vi "Setup NI cDAQ-9188.vi"(8 "error in":errorcluster, 9 "Samples per Channel":i32=100, 10 "Sample Rate":dbl=100000.0, 11 "Physical Channels":string) -> (0 "error out":errorcluster, 2 "Counter Task":refnum<k21>, 3 "AI Voltage Task":refnum<k21>)   [LabVIEW 2013, in "Breakdown Acoustics Controls.lvlib"]
uses:
  <vilib>/DAQmx/create/channels.llb/DAQmx Create Channel (AI-Voltage-Basic).vi
  <vilib>/DAQmx/configure/timing.llb/DAQmx Timing (Sample Clock).vi
  <vilib>/DAQmx/create/channels.llb/DAQmx Create Channel (CO-Pulse Generation-Frequency).vi
  <vilib>/DAQmx/configure/timing.llb/DAQmx Timing (Implicit).vi
  <vilib>/DAQmx/configure/trigger.llb/DAQmx Start Trigger (Digital Edge).vi
  Breakdown Acoustics Controls.lvlib
  <resource>/objmgr/daqmx.rc
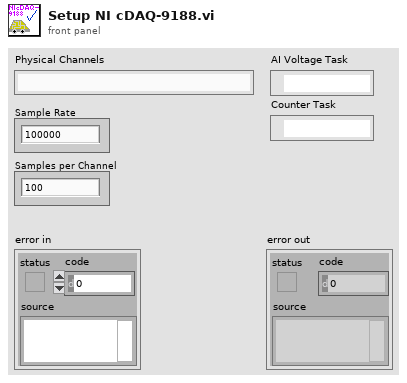
[diagram p1: front panel]
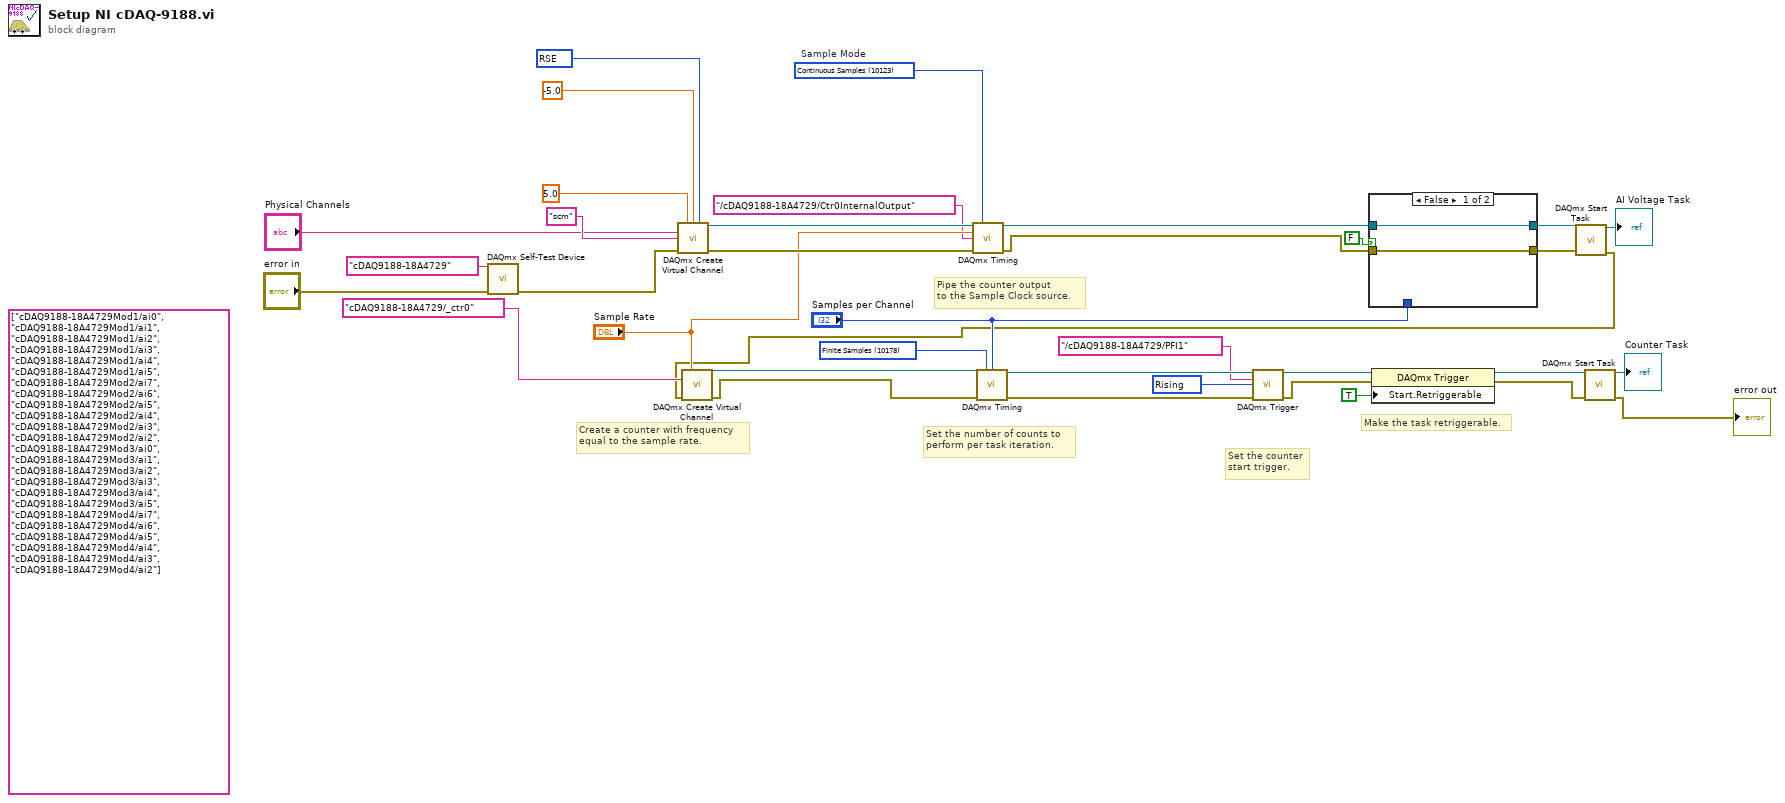
[diagram p0: block diagram]
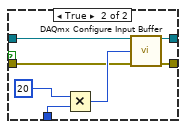
[diagram p2: hidden frame]
diagram:
  w14 = 10280 items=["Rising"=10280, "Falling"=10171] ("edge")
  w33 = 10083 items=["default"=-1, "RSE"=10083, "NRSE"=10078, "Differential"=10106, "Pseudodifferential"=12529] ("Terminal Configuration")
  w29 = 10178 items=["Finite Samples"=10178, "Continuous Samples"=10123, "Hardware Timed Single Point"=12522] ("sample mode")
  (unwired) tag[] ["cDAQ9188-18A4729Mod1/ai0", "cDAQ9188-18A4729Mod1/ai1", "cDAQ9188-18A4729Mod1/ai2", "cDAQ9188-18A4729Mod1/ai3", "cDAQ9188-18A4729Mod1/ai4", "cDAQ9188-18A4729Mod1/ai5", "cDAQ9188-18A4729Mod2/ai7", "cDAQ9188-18A4729Mod2/ai6", "cDAQ9188-18A4729Mod2/ai5", "cDAQ9188-18A4729Mod2/ai4", "cDAQ9188-18A4729Mod2/ai3", "cDAQ9188-18A4729Mod2/ai2", "cDAQ9188-18A4729Mod3/ai0", "cDAQ9188-18A4729Mod3/ai1", "cDAQ9188-18A4729Mod3/ai2", "cDAQ9188-18A4729Mod3/ai3", "cDAQ9188-18A4729Mod3/ai4", "cDAQ9188-18A4729Mod3/ai5", "cDAQ9188-18A4729Mod4/ai7", "cDAQ9188-18A4729Mod4/ai6", "cDAQ9188-18A4729Mod4/ai5", "cDAQ9188-18A4729Mod4/ai4", "cDAQ9188-18A4729Mod4/ai3", "cDAQ9188-18A4729Mod4/ai2"]
  w36 = 10123 items=["Finite Samples"=10178, "Continuous Samples"=10123, "Hardware Timed Single Point"=12522]  # Sample Mode
  # "Set the counter\nstart trigger."
  # "Make the task retriggerable."
  # "Set the number of counts to\nperform per task iteration."
  # "Pipe the counter output\nto the Sample Clock source."
  # "Create a counter with frequency\nequal to the sample rate."
  n1 = call <vilib>:"DAQmx Self-Test Device.vi"("device in"=tag "cDAQ9188-18A4729", "error in"="error in") -> ("error out"=w7:errorcluster)  [unwired: 13 in]
  n2 = call-poly <vilib>:"DAQmx Create Virtual Channel.vi"("maximum value"=5.0 ("Max Voltage"), "minimum value"=-5.0 ("Min Voltage"), "input terminal configuration"=w33, "physical channels"="Physical Channels", "name to assign"="scm", "error in"=w7) -> ("task out"=w34:refnum<k21>, "error out"=w35:errorcluster)  [unwired: 8 in]
  n3 = call-poly <vilib>:"DAQmx Timing.vi"("task/channels in"=w34, "sample mode"=w36, "rate"="Sample Rate", "source"=tag "/cDAQ9188-18A4729/Ctr0InternalOutput" ("CO.Pulse.Term"), "error in"=w35) -> ("task out"=w2:refnum<k21>, "error out"=w1:errorcluster)  [unwired: 9 in]
  n4 = case shown="False" FALSE {
    tunnel: w2 -> [w38 w44]
    tunnel: w1 -> [w37 w43]
    tunnel: [w38 w42] -> w19
    tunnel: [w37 w41] -> w18
    tunnel: "Samples per Channel" -> [_ w39]
    frame False {
    }
    frame True {
      n5 = Multiply(x=u32 20, y=w39) -> (x*y=w45:u32)
      n6 = call <vilib>:"DAQmx Configure Input Buffer.vi"("task/channels in"=w44, "buffer size (in samples per channel)"=w45, "error in"=w43) -> ("task out"=w42:refnum<k21>, "error out"=w41:errorcluster)  [unwired: 11 in]
    }
  }
  n7 = call <vilib>:"DAQmx Start Task.vi"("task/channels in"=w19, "error in"=w18) -> ("task out"=→"AI Voltage Task":refnum<k21>, "error out"=w11:errorcluster)  [unwired: 12 in]
  n8 = call-poly <vilib>:"DAQmx Create Virtual Channel.vi"("frequency"="Sample Rate", "counter"=tag "cDAQ9188-18A4729/_ctr0" ("Counter*"), "error in"=w11) -> ("task out"=w13:refnum<k21>, "error out"=w12:errorcluster)  [unwired: 11 in]
  n9 = call-poly <vilib>:"DAQmx Timing.vi"("task/channels in"=w13, "sample mode"=w29, "samples per channel"="Samples per Channel", "error in"=w12) -> ("task out"=w27:refnum<k21>, "error out"=w26:errorcluster)  [unwired: 10 in]
  n10 = call-poly <vilib>:"DAQmx Trigger.vi"("task/channels in"=w27, "source"=tag "/cDAQ9188-18A4729/PFI1" ("Trigger Source"), "edge"=w14, "error in"=w26) -> ("task out"=w25:refnum<k21>, "error out"=w24:errorcluster)  [unwired: 10 in]
  n11 = property class="DAQmx Trigger"(reference=w25, error in=w24, "Start.Retriggerable"=TRUE) -> (reference out=w21:refnum<k21>, error out=w20:errorcluster)
  n12 = call <vilib>:"DAQmx Start Task.vi"("task/channels in"=w21, "error in"=w20) -> ("task out"=→"Counter Task":refnum<k21>, "error out"=→"error out":errorcluster)  [unwired: 12 in]
